vi "Replace Multiple Wheels in Steering Frame.vi"(5 "x positions":dbl[](array[numeric]), 6 "frame angles (rad)":dbl[](array[numeric]), 7 "y positions":dbl[](array[numeric]), 8 "error in (no error)":errorcluster, 9 "wheels":refnum<class "NI_Robotics_Wheel.lvclass">[](array[class]), 10 "wheel indexes":i32[](array[numeric]), 11 "steering frame in":refnum<class "NI_Robotics_Steering Frame.lvclass">) -> (0 "error out":errorcluster, 1 "found?":bool[](array[boolean]), 3 "steering frame out":refnum<class "NI_Robotics_Steering Frame.lvclass">)   [LabVIEW 2017, in "NI_Robotics_Steering Frame.lvclass"]
doc: "Replaces wheels in <B>steering frame in</B> with the wheels you specify. You must manually select the polymorphic instance to use."
uses:
  <vilib>/robotics/Steering/Steering Frame/NI_Robotics_Steering Frame.lvclass
  <vilib>/robotics/Steering/Wheel/NI_Robotics_Wheel.lvclass
  <vilib>/robotics/Steering/Steering Frame/NI_Robotics_Steering Frame.lvclass/NI_Robotics_Steering Frame.ctl
  <vilib>/robotics/Steering/Wheel/NI_Robotics_Wheel.lvclass/NI_Robotics_Wheel.ctl
  <vilib>/robotics/Steering/Wheel/Update Steering to Wheel Frame Transform.vi
  <vilib>/Analysis/coordinate.llb/Wrap Angle.vi
  <vilib>/Analysis/coordinate.llb/Wrap Angle (scalar).vi
  <vilib>/robotics/Steering/Wheel/Get Wheel Name.vi
  <vilib>/robotics/Utilities/NI_Robotics Utilities.lvlib
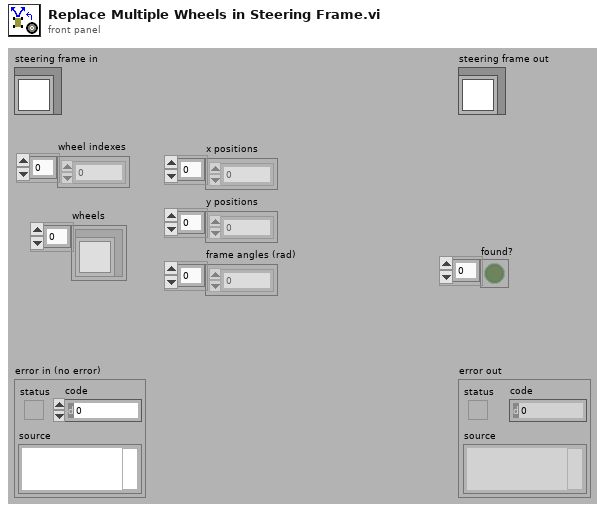
[diagram p1: front panel]
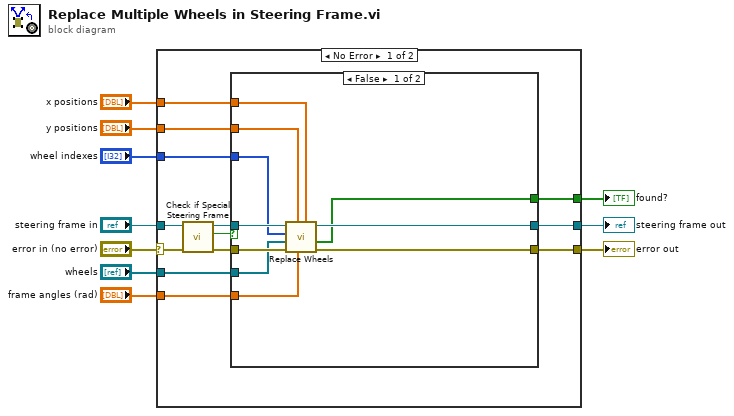
[diagram p0: block diagram]
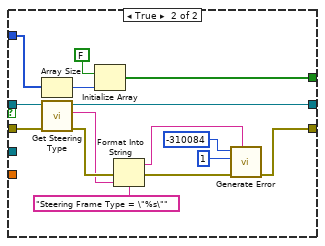
[diagram p2: hidden frame]
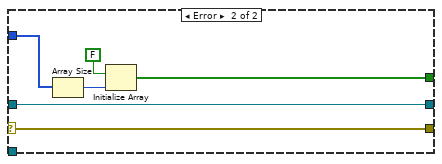
[diagram p3: hidden frame]
diagram:
  n1 = case shown="No Error" "error in (no error)" {
    selector: "error in (no error)" -> [w14 w54]
    tunnel: [w11 w54] -> w9
    tunnel: [w22 w53] -> w7
    tunnel: "steering frame in" -> [w16 w53]
    tunnel: "wheel indexes" -> [w21 w49]
    tunnel: "wheels" -> [w23 _]
    tunnel: [w20 w50] -> w5
    tunnel: "x positions" -> [w19 _]
    tunnel: "y positions" -> [w18 _]
    tunnel: "frame angles (rad)" -> [w17 _]
    frame No Error {
      n2 = call-dynamic "Check if Special Steering Frame.vi"("error in (no error)"=w14, "steering frame in"=w16) -> ("error out"=w13:errorcluster, "special?"=w12:bool, "steering frame out"=w15:refnum<class "NI_Robotics_Steering Frame.lvclass">)  [unwired: 7 in]
      n3 = case shown="False" w12 {
        tunnel: w23 -> [w31 _]
        tunnel: [w26 w44] -> w22
        tunnel: w21 -> [w30 w34]
        tunnel: [w24 w35] -> w20
        tunnel: w19 -> [w28 _]
        tunnel: w18 -> [w27 _]
        tunnel: w17 -> [w29 _]
        tunnel: w15 -> [w33 w45]
        tunnel: w13 -> [w32 w43]
        tunnel: [w25 w46] -> w11
        frame False {
          n4 = call <vilib>:"Replace Wheels.vi"("x positions"=w28, "frame angles (rad)"=w29, "y positions"=w27, "error in (no error)"=w32, "wheels"=w31, "wheel indexes"=w30, "steering frame in"=w33) -> ("error out"=w25:errorcluster, "found?"=w24:bool[], "steering frame out"=w26:refnum<class "NI_Robotics_Steering Frame.lvclass">)  [unwired: 2 in]
        }
        frame True {
          n5 = Array Size(array=w34) -> (size(s)=w37:i32)
          n6 = call-dynamic "Get Steering Type.vi"("error in (no error)"=w43, "steering frame in"=w45) -> ("error out"=w42:errorcluster, "steering type"=w40:string, "steering frame out"=w44:refnum<class "NI_Robotics_Steering Frame.lvclass">)  [unwired: 7 in]
          n7 = Initialize Array(FALSE, w37) -> (w35:bool[])
          n8 = Format Into String(format string="Steering Frame Type = \"%s\"", error in=w42, w40) -> (resulting string=w39:string, error out=w41:errorcluster)  [unwired: 1 in]
          n9 = call <vilib>:"Generate Error.vi"("<append> (\"\")"=w39, "error in (no error)"=w41, "chain levels to remove (1)"=1, "code"=-310084) -> ("error out"=w46:errorcluster)  [unwired: 7 in]
        }
      }
    }
    frame Error {
      n10 = Array Size(array=w49) -> (size(s)=w52:i32)
      n11 = Initialize Array(FALSE, w52) -> (w50:bool[])
    }
  }
  "error out" <- w9
  "steering frame out" <- w7
  "found?" <- w5
